vi "CRYRub & Buzz weight function.vi"(10 "Numeric":i32=2048) -> (3 "ear wight":dbl[](array[numeric]))   [LabVIEW 2013]
panel:
  out "XY Graph":cluster{dbl[], dbl[]}(graph) caption="Stimulus_Ear_Graph"
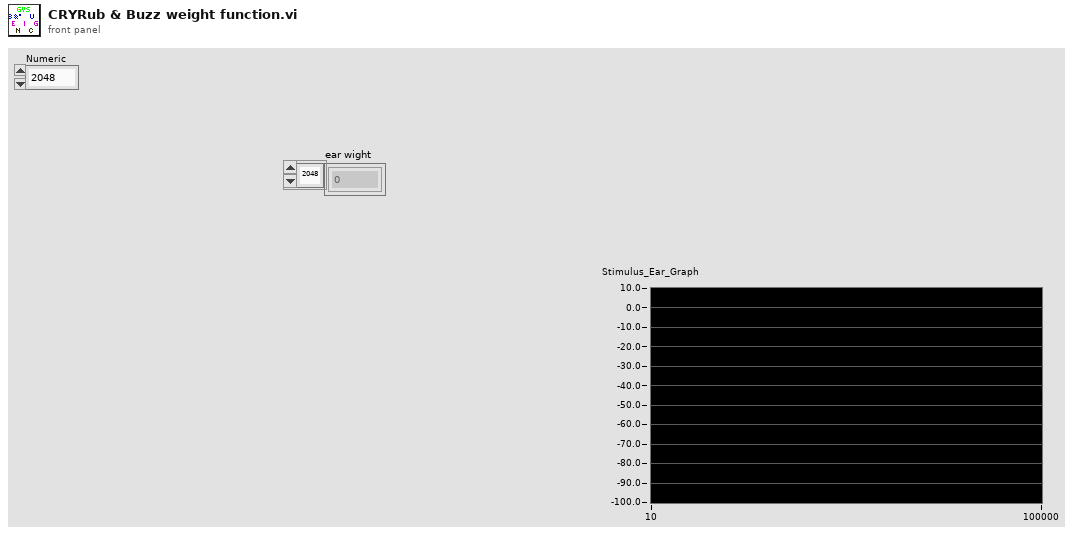
[diagram p1: front panel]
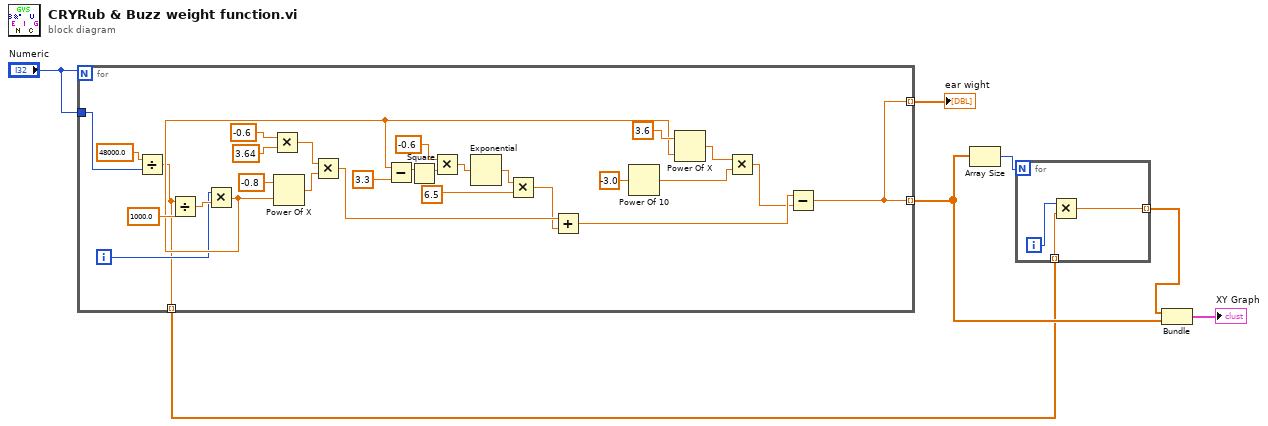
[diagram p0: block diagram]
diagram:
  n1 = for {
    N: "Numeric" -> [_]
    tunnel: [w11] -> w7 mode=indexing
    tunnel: [w11] -> w6 mode=indexing
    tunnel: "Numeric" -> [w8]
    tunnel: [w9] -> w4 mode=indexing
    i -> [w12]
    n2 = Divide(x=48000.0, y=w8) -> (x/y=w9:dbl)
    n3 = Divide(x=w9, y=1000.0) -> (x/y=w22:dbl)
    n4 = Multiply(x=w12, y=w22) -> (x*y=w13:dbl)
    n5 = Multiply(x=-0.6, y=3.64) -> (x*y=w30:dbl)
    n6 = Power Of X(1:w13, 2:-0.8 ("y")) -> (0:w31:dbl)
    n7 = Multiply(x=w30, y=w31) -> (x*y=w16:dbl)
    n8 = Subtract(x=w13, y=3.3) -> (x-y=w27:dbl)
    n9 = Square(x=w27) -> (x^2=w26:dbl)
    n10 = Multiply(x=-0.6, y=w26) -> (x*y=w25:dbl)
    n11 = Exponential(1:w25) -> (0:w24:dbl)
    n12 = Multiply(x=w24, y=6.5) -> (x*y=w15:dbl)
    n13 = Add(x=w16, y=w15) -> (x+y=w17:dbl)
    n14 = Power Of 10(x=-3.0) -> (10^x=w18:dbl)
    n15 = Power Of X(1:w13, 2:3.6) -> (0:w19:dbl)
    n16 = Multiply(x=w19, y=w18) -> (x*y=w14:dbl)
    n17 = Subtract(x=w17, y=w14) -> (x-y=w11:dbl)
  }
  "ear wight" <- w6
  n18 = Array Size(array=w7) -> (size(s)=w2:i32)
  n19 = for {
    N: w2 -> [_]
    tunnel: [w37] -> w1 mode=indexing
    tunnel: w4 -> [w36] mode=indexing
    i -> [w38]
    n20 = Multiply(x=w38, y=w36) -> (x*y=w37:dbl)
  }
  n21 = Bundle(w1, w7) -> (→"XY Graph":cluster{dbl[], dbl[]})  [unwired: 1 out]
